vi "Turret_Accumulator.vi"(1 "Position (Raw Sensor Units)":i32) -> (0 "Turret_Wraparound":i32)   [LabVIEW 2019]
uses:
  Globals/Turret_Globals.vi
panel:
  in  "ticks per revolution":i32=4096
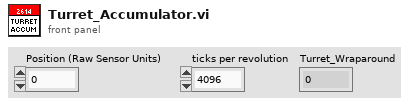
[diagram p1: front panel]
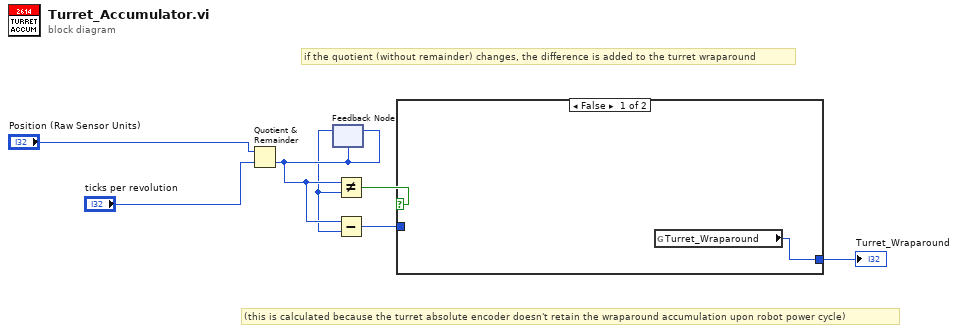
[diagram p0: block diagram]
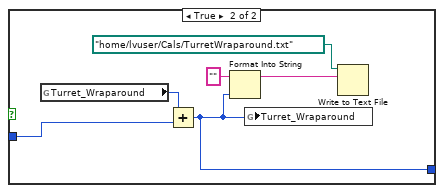
[diagram p2: hidden frame]
diagram:
  # "(this is calculated because the turret absolute encoder doesn't retain the wraparound accumulation upon robot power cycle)"
  # "if the quotient (without remainder) changes, the difference is added to the turret wraparound"
  n1 = Quotient & Remainder(x="Position (Raw Sensor Units)", y="ticks per revolution") -> (floor(x/y)=w3:i32)  [unwired: 1 out]
  n2 = feedback-in #1(w3) -> ()
  n3 = feedback #1(w3) -> (w2:i32)
  n4 = Not Equal?(x=w3, y=w2) -> (x != y?=w5:bool)
  n5 = Subtract(x=w3, y=w2) -> (x-y=w4:i32)
  n6 = case shown="False" w5 {
    tunnel: w4 -> [_ w13]
    tunnel: [w8 w9] -> w1
    frame False {
      n7 = global read "Turret_Globals.vi" "Turret_Wraparound"() -> (w8:i32)
    }
    frame True {
      n8 = global read "Turret_Globals.vi" "Turret_Wraparound"() -> (w14:i32)
      n9 = Add(x=w14, y=w13) -> (x+y=w9:i32)
      n10 = Format Into String(initial string="", w9) -> (resulting string=w12:string)  [unwired: 2 in, 1 out]
      n11 = global write "Turret_Globals.vi" "Turret_Wraparound"(w9) -> ()
      n12 = Write to Text File(file (use dialog)=path "/home/lvuser/Cals/TurretWraparound.txt", text=w12) -> ()  [unwired: 2 in, 3 out]
    }
  }
  "Turret_Wraparound" <- w1
